vi "Image.vi"(2 "XRef":refnum<vi>, 3 "State In":T1) -> (0 "Image":picture)   [LabVIEW 2012, in "OpenG Reverse 2D Array.xnode"]
uses:
  OpenG Reverse 2D Array.xnode
  State.ctl
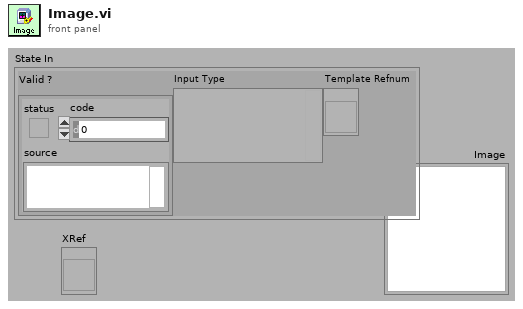
[diagram p1: front panel]
types:
  T1 = typedef "OpenG Reverse 2D Array.xnode/State.ctl" = cluster{"Valid ?":errorcluster, "Input Type":variant, "Template Refnum":refnum<vi>}
  T2 = typedef "imagedata.ctl" = cluster{"image type":i32, "image depth":i32, "image":u8[], "mask":u8[], "colors":u32[], "Rectangle":cluster{"left":i16, "top":i16, "right":i16, "bottom":i16}}
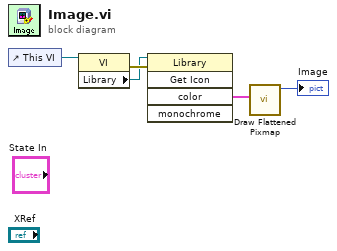
[diagram p0: block diagram]
diagram:
  n1 = control-ref of="This VI"() -> (w4:refnum<vi>)
  n2 = property class="VI"(reference=w4) -> (error out=w3:errorcluster, "Library"=w2:refnum<vi>)  [unwired: 1 in, 1 out]
  n3 = invoke class="Library" method="Get Icon"(reference=w2, error in=w3) -> ("color"=w1:T2)  [unwired: 3 in, 4 out]
  n4 = call <vilib>:"Draw Flattened Pixmap.vi"("image data"=w1) -> ("new picture"=→"Image":picture)  [unwired: 1 in, 7 out]
